vi "SubVI_Camera_Test.vi"(4 "V Width":i32 min=4 max=2048 step=4, 5 "V Offset":i32 min=0 max=0 step=4, 6 "H Width":i32 min=4 max=2048 step=4, 7 "H Offset":i32 min=0 max=0 step=4, 8 "error in":errorcluster, 9 "Exposure Time IN":dbl=0.1 format="%#_13g", 10 "Binning":i32(ring)=1 items=["1x1"=1, "2x2"=2, "4x4"=4], 11 "Menu":T3) -> (0 "error out":errorcluster, 1 "Image":u16[][](graph), 2 "Status":u32, 3 "Temps mesuré ms":u32)   [LabVIEW 2014]
uses:
  Control 1.ctl
  <vilib>/Utility/miscctls.llb/LVMinMaxIncTypeDef.ctl
panel:
  out "Sub Region":T2 {"V Size"."Value" min=0 max=0 step=4; "H Size"."Value" min=0 max=0 step=4; "V Offset"."Value" min=0 max=0 step=4; "H Offset"."Value" min=0 max=0 step=4}
  out "Exposure Time OUT Init S":dbl
  in  "Exposure Time IN Init":dbl=0.1 format="%#_13g"
  out "Exposure Time OUT Init mS":dbl
  out "Exposure Time out":dbl
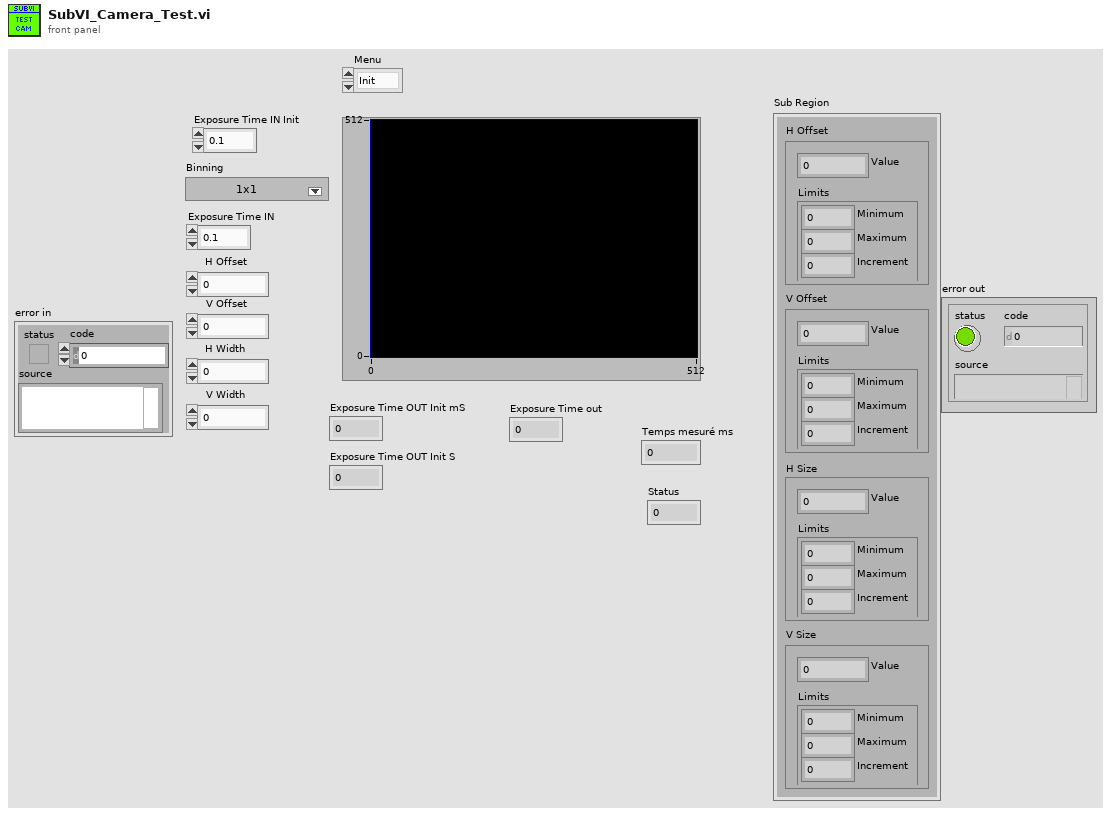
[diagram p1: front panel]
types:
  T1 = typedef "LVMinMaxIncTypeDef.ctl" = cluster{"Minimum":dbl, "Maximum":dbl, "Increment":dbl}
  T2 = cluster{"H Offset":cluster{"Value":i32, "Limits":T1}, "V Offset":cluster{"Value":i32, "Limits":T1}, "H Size":cluster{"Value":i32, "Limits":T1}, "V Size":cluster{"Value":i32, "Limits":T1}}
  T3 = typedef "Control 1.ctl" = enum16{"Init", "Statut", "Binning", "Width", "Exposure Time", "Rep", "Capture", "Stop"}
  T4 = cluster{"H Offset":i32, "V Offset":i32, "H Width":i32, "V Width":i32}
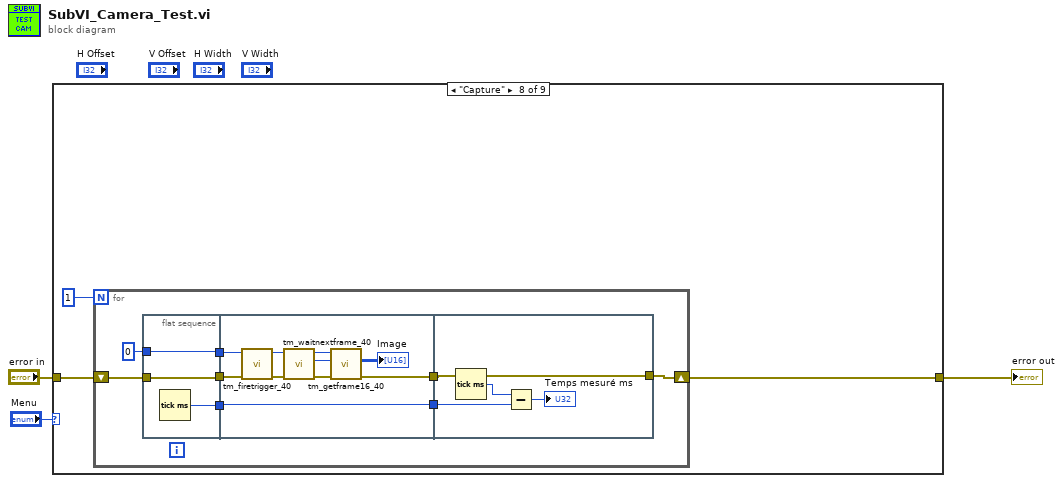
[diagram p0: block diagram]
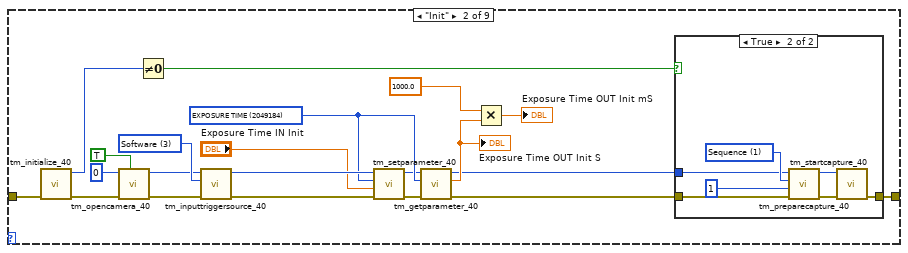
[diagram p3: hidden frame]
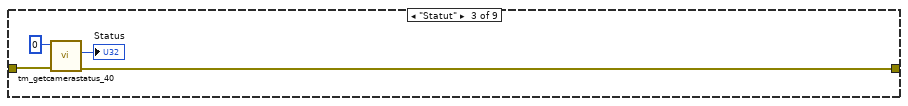
[diagram p5: hidden frame]
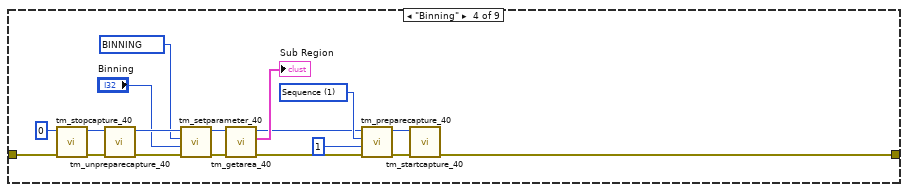
[diagram p6: hidden frame]
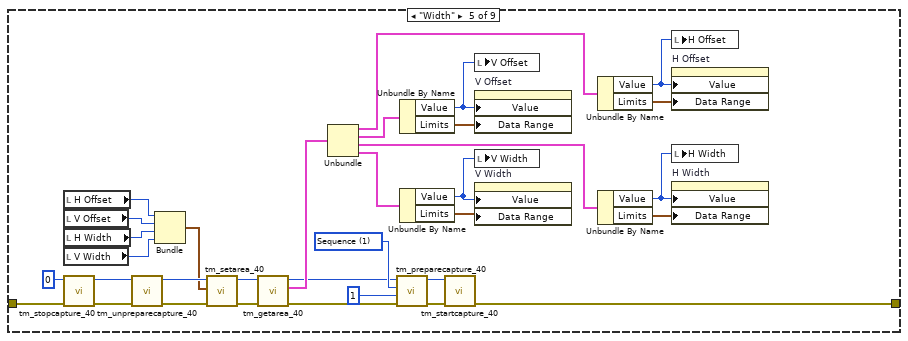
[diagram p7: hidden frame]
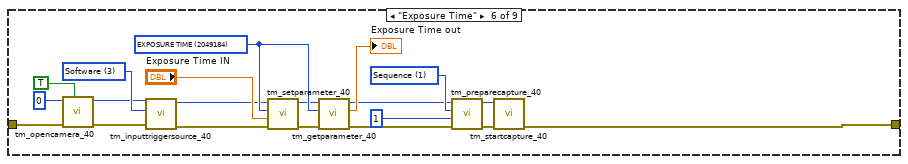
[diagram p8: hidden frame]
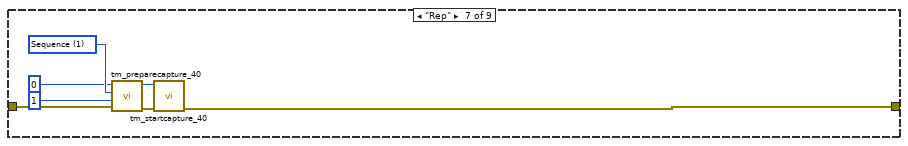
[diagram p9: hidden frame]
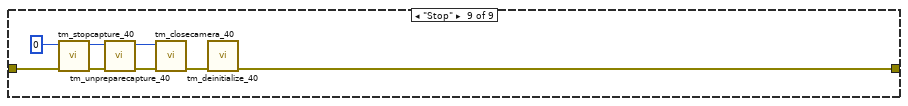
[diagram p10: hidden frame]
diagram:
  n1 = case shown="\"Capture\"" "Menu" {
    tunnel: "error in" -> [w4 w25 w35 w48 w64 w94 w112 w118 w146]
    tunnel: [w4 w5 w37 w38 w57 w98 w111 w117 w144] -> w1
    frame Default {
    }
    frame "Init" {
      w18 = 3 items=["Internal"=1, "External"=2, "Software"=3, "Master Pulse"=4] ("Source")
      w14 = u32 2049184 items=["SENSOR MODE"=4212128, "SENSOR MODE LINE BUNDLE HEIGHT"=4212192, "READOUT DIRECTION"=4211904, "BIT PER CHANNEL"=4342976, "EXPOSURE TIME"=2049184, "CONTRAST GAIN"=3163312, "BINNING"=4215968, "TIMING READOUT TIME"=4223904, "INTERNAL FRAME RATE"=4225952, "INTERNAL FRAME INTERVAL"=4225968, "INTERNAL LINE SPEED"=4226000, "IMAGE WIDTH"=4343200, "IMAGE HEIGHT"=4343216, "IMAGE ROWBYTES"=4343232, "IMAGE FRAMEBYTES"=4343248, "IMAGE PIXEL TYPE"=4343296] ("Parameter")
      n2 = call <userlib>:"tm_initialize_40.vi"("error in (no error)"=w25) -> ("error out"=w22:errorcluster, "Number Of Cameras"=w24:u32)  [unwired: 7 in, 2 out]
      n3 = call <userlib>:"tm_opencamera_40.vi"("Force Open"=TRUE, "error in (no error)"=w22, "Camera Index"=u32 0) -> ("error out"=w10:errorcluster, "Handle out"=w9:u32)  [unwired: 6 in, 1 out]
      n4 = Not Equal To 0?(x=w24) -> (x != 0?=w8:bool)
      n5 = call <userlib>:"tm_inputtriggersource_40.vi"("error in (no error)"=w10, "Source"=w18, "Handle in"=w9) -> ("error out"=w19:errorcluster, "Handle out"=w20:u32)  [unwired: 7 in]
      n6 = call <userlib>:"tm_setparameter_40.vi"("error in (no error)"=w19, "Value in"="Exposure Time IN Init", "Parameter"=w14, "Handle in"=w20) -> ("error out"=w12:errorcluster, "Handle out"=w13:u32)  [unwired: 6 in]
      n7 = call <userlib>:"tm_getparameter_40.vi"("error in (no error)"=w12, "Parameter"=w14, "Handle in"=w13) -> ("error out"=w7:errorcluster, "Value out"=w15:dbl, "Handle out"=w6:u32)  [unwired: 6 in]
      "Exposure Time OUT Init S" <- w15
      n8 = Multiply(x=1000.0, y=w15) -> (x*y=→"Exposure Time OUT Init mS":dbl)
      n9 = case shown="True" w8 {
        tunnel: w7 -> [w26 w28]
        tunnel: w6 -> [_ w29]
        tunnel: [w26 w27] -> w5
        frame False {
        }
        frame True {
          w33 = 1 items=["Snap", "Sequence"] ("Capture mode")
          n10 = call <userlib>:"tm_preparecapture_40.vi"("error in (no error)"=w28, "Frames"=1, "Capture mode"=w33, "Handle in"=w29) -> ("error out"=w31:errorcluster, "Handle out"=w32:u32)  [unwired: 4 in, 2 out]
          n11 = call <userlib>:"tm_startcapture_40.vi"("error in (no error)"=w31, "Handle in"=w32) -> ("error out"=w27:errorcluster)  [unwired: 8 in, 1 out]
        }
      }
    }
    frame "Statut" {
      n12 = call <userlib>:"tm_getcamerastatus_40.vi"("error in (no error)"=w35, "Handle in"=u32 0) -> ("error out"=w37:errorcluster, "Status"=→"Status":i32)  [unwired: 7 in, 1 out]
    }
    frame "Binning" {
      w41 = 1 items=["Snap", "Sequence"] ("Capture mode")
      w52 = u32 4215968 items=["BINNING"=4215968, "BITS PER CHANNEL"=2, "ACTIVE VIEW INDEX"=3, "CCD MODE"=4, "SENSOR MODE"=5, "READOUT MODE"=6, "EXPOSURE TIME"=7, "CONTRAST GAIN"=8, "CONTRAST OFFSET"=9, "LIGHT MODE"=10, "SENSITIVITY"=11, "WHITE BALANCE"=12, "PHOTON IMAGING MODE"=13, "HIGH DYNAMIC RANGE MODE"=14, "TRIGGER SOURCE"=15, "TRIGGER ACTIVE"=16, "TRIGGER MODE"=17, "TRIGGER POLARITY"=18, "TRIGGER GLOBAL EXPOSURE"=19, "FIRST TRIGGER BEHAVIOR"=20, "TRIGGER TIMES"=21, "OUTPUT TRIGGER POLARITY"=22, "OUTPUT TRIGGER DELAY"=23, "OUTPUT TRIGGER PERIOD"=24, "TEMPERATURE"=25, "TEMPERATURE TARGET"=26, "SENSOR COOLER FAN"=27, "MECHANICAL SHUTTER"=28, "BACK FOCUS POSITION"=29, "FRAMEBUNDLE MODE"=30, "FRAMEBUNDLE NUMBER"=31, "LINEBUNDLE HEIGHT"=32, "TRIGGER CONNECTOR"=33, "IMAGE PIXEL TYPE"=34, "OUTPUT TRIGGER KIND"=35, "READOUT DIRECTION"=36, "CHANNEL SYNC"=37] ("Parameter")
      n13 = call <userlib>:"tm_stopcapture_40.vi"("error in (no error)"=w48, "Handle in"=u32 0) -> ("error out"=w50:errorcluster, "Handle out"=w49:u32)  [unwired: 8 in]
      n14 = call <userlib>:"tm_unpreparecapture_40.vi"("error in (no error)"=w50, "Handle in"=w49) -> ("error out"=w51:errorcluster, "Handle out"=w53:u32)  [unwired: 8 in]
      n15 = call <userlib>:"tm_setparameter_40.vi"("error in (no error)"=w51, "Value in"="Binning", "Parameter"=w52, "Handle in"=w53) -> ("error out"=w55:errorcluster, "Handle out"=w54:u32)  [unwired: 6 in]
      n16 = call <userlib>:"tm_getarea_40.vi"("error in (no error)"=w55, "Handle in"=w54) -> ("error out"=w39:errorcluster, "Sub Region"=→"Sub Region":T2, "Handle out"=w40:u32)  [unwired: 7 in]
      n17 = call <userlib>:"tm_preparecapture_40.vi"("error in (no error)"=w39, "Frames"=1, "Capture mode"=w41, "Handle in"=w40) -> ("error out"=w43:errorcluster, "Handle out"=w42:u32)  [unwired: 4 in, 2 out]
      n18 = call <userlib>:"tm_startcapture_40.vi"("error in (no error)"=w43, "Handle in"=w42) -> ("error out"=w38:errorcluster)  [unwired: 8 in, 1 out]
    }
    frame "Width" {
      w62 = 1 items=["Snap", "Sequence"] ("Capture mode")
      n19 = local read "H Offset"() -> (w82:i32)
      n20 = local read "V Offset"() -> (w81:i32)
      n21 = local read "H Width"() -> (w80:i32)
      n22 = local read "V Width"() -> (w79:i32)
      n23 = call <userlib>:"tm_stopcapture_40.vi"("error in (no error)"=w64, "Handle in"=u32 0) -> ("error out"=w84:errorcluster, "Handle out"=w83:u32)  [unwired: 8 in]
      n24 = call <userlib>:"tm_unpreparecapture_40.vi"("error in (no error)"=w84, "Handle in"=w83) -> ("error out"=w86:errorcluster, "Handle out"=w85:u32)  [unwired: 8 in]
      n25 = Bundle("H Offset"=w82, "V Offset"=w81, "H Width"=w80, "V Width"=w79) -> (w78:T4)  [unwired: 1 in]
      n26 = call <userlib>:"tm_setarea_40.vi"("error in (no error)"=w86, "Sub Region"=w78, "Handle in"=w85) -> ("error out"=w88:errorcluster, "Handle out"=w87:u32)  [unwired: 7 in]
      n27 = call <userlib>:"tm_getarea_40.vi"("error in (no error)"=w88, "Handle in"=w87) -> ("error out"=w58:errorcluster, "Sub Region"=w69:T2, "Handle out"=w56:u32)  [unwired: 7 in]
      n28 = Unbundle(w69) -> ("H Offset"=w77:cluster{"Value":i32, "Limits":T1}, "V Offset"=w76:cluster{"Value":i32, "Limits":T1}, "H Size"=w75:cluster{"Value":i32, "Limits":T1}, "V Size"=w74:cluster{"Value":i32, "Limits":T1})
      n29 = call <userlib>:"tm_preparecapture_40.vi"("error in (no error)"=w58, "Frames"=1, "Capture mode"=w62, "Handle in"=w56) -> ("error out"=w60:errorcluster, "Handle out"=w61:u32)  [unwired: 4 in, 2 out]
      n30 = Unbundle By Name(w76) -> ("Value"=w67:i32, "Limits"=w72:T1)
      n31 = Unbundle By Name(w74) -> ("Value"=w65:i32, "Limits"=w70:T1)
      n32 = call <userlib>:"tm_startcapture_40.vi"("error in (no error)"=w60, "Handle in"=w61) -> ("error out"=w57:errorcluster)  [unwired: 8 in, 1 out]
      n33 = local write "V Offset"(w67) -> ()
      n34 = property on="V Offset" class="DigNum (strict)"("Value"=w67, "Data Range"=w72) -> ()  [unwired: 2 in, 2 out]
      n35 = local write "V Width"(w65) -> ()
      n36 = property on="V Width" class="DigNum (strict)"("Value"=w65, "Data Range"=w70) -> ()  [unwired: 2 in, 2 out]
      n37 = Unbundle By Name(w77) -> ("Value"=w68:i32, "Limits"=w73:T1)
      n38 = Unbundle By Name(w75) -> ("Value"=w66:i32, "Limits"=w71:T1)
      n39 = local write "H Offset"(w68) -> ()
      n40 = property on="H Offset" class="DigNum (strict)"("Value"=w68, "Data Range"=w73) -> ()  [unwired: 2 in, 2 out]
      n41 = local write "H Width"(w66) -> ()
      n42 = property on="H Width" class="DigNum (strict)"("Value"=w66, "Data Range"=w71) -> ()  [unwired: 2 in, 2 out]
    }
    frame "Exposure Time" {
      w93 = 3 items=["Internal"=1, "External"=2, "Software"=3, "Master Pulse"=4] ("Source")
      w103 = 1 items=["Snap", "Sequence"] ("Capture mode")
      w108 = u32 2049184 items=["SENSOR MODE"=4212128, "SENSOR MODE LINE BUNDLE HEIGHT"=4212192, "READOUT DIRECTION"=4211904, "BIT PER CHANNEL"=4342976, "EXPOSURE TIME"=2049184, "CONTRAST GAIN"=3163312, "BINNING"=4215968, "TIMING READOUT TIME"=4223904, "INTERNAL FRAME RATE"=4225952, "INTERNAL FRAME INTERVAL"=4225968, "INTERNAL LINE SPEED"=4226000, "IMAGE WIDTH"=4343200, "IMAGE HEIGHT"=4343216, "IMAGE ROWBYTES"=4343232, "IMAGE FRAMEBYTES"=4343248, "IMAGE PIXEL TYPE"=4343296] ("Parameter")
      n43 = call <userlib>:"tm_opencamera_40.vi"("Force Open"=TRUE, "error in (no error)"=w94, "Camera Index"=u32 0) -> ("error out"=w89:errorcluster, "Handle out"=w92:u32)  [unwired: 6 in, 1 out]
      n44 = call <userlib>:"tm_inputtriggersource_40.vi"("error in (no error)"=w89, "Source"=w93, "Handle in"=w92) -> ("error out"=w90:errorcluster, "Handle out"=w91:u32)  [unwired: 7 in]
      n45 = call <userlib>:"tm_setparameter_40.vi"("error in (no error)"=w90, "Value in"="Exposure Time IN", "Parameter"=w108, "Handle in"=w91) -> ("error out"=w106:errorcluster, "Handle out"=w107:u32)  [unwired: 6 in]
      n46 = call <userlib>:"tm_getparameter_40.vi"("error in (no error)"=w106, "Parameter"=w108, "Handle in"=w107) -> ("error out"=w99:errorcluster, "Value out"=→"Exposure Time out":dbl, "Handle out"=w97:u32)  [unwired: 6 in]
      n47 = call <userlib>:"tm_preparecapture_40.vi"("error in (no error)"=w99, "Frames"=1, "Capture mode"=w103, "Handle in"=w97) -> ("error out"=w101:errorcluster, "Handle out"=w100:u32)  [unwired: 4 in, 2 out]
      n48 = call <userlib>:"tm_startcapture_40.vi"("error in (no error)"=w101, "Handle in"=w100) -> ("error out"=w98:errorcluster)  [unwired: 8 in, 1 out]
    }
    frame "Rep" {
      w110 = 1 items=["Snap", "Sequence"] ("Capture mode")
      n49 = call <userlib>:"tm_preparecapture_40.vi"("error in (no error)"=w112, "Frames"=1, "Capture mode"=w110, "Handle in"=u32 0) -> ("error out"=w114:errorcluster, "Handle out"=w115:u32)  [unwired: 4 in, 2 out]
      n50 = call <userlib>:"tm_startcapture_40.vi"("error in (no error)"=w114, "Handle in"=w115) -> ("error out"=w111:errorcluster)  [unwired: 8 in, 1 out]
    }
    frame "Capture" {
      n51 = for {
        N: 1 -> [_]
        shift-right: [w123] -> w117
        shift-left: w118 -> [w119]
        n52 = flat-sequence {
          tunnel: [w129] -> w126
          tunnel: [w128] -> w122
          tunnel: [w127] -> w121
          tunnel: u32 0 ("Handle out") -> [w128]
          tunnel: w119 -> [w127]
          tunnel: [w130] -> w125
          tunnel: [w139] -> w124
          tunnel: w126 -> [w139]
          tunnel: w122 -> [w133]
          tunnel: w121 -> [w132]
          tunnel: [w140] -> w123
          tunnel: w125 -> [w140]
          tunnel: w124 -> [w141]
          frame #0 {
            n53 = Tick Count (ms)() -> (millisecond timer value=w129:u32)
          }
          frame #1 {
            n54 = call <userlib>:"tm_firetrigger_40.vi"("error in (no error)"=w132, "Handle in"=w133) -> ("error out"=w135:errorcluster, "Handle out"=w134:u32)  [unwired: 8 in]
            n55 = call <userlib>:"tm_waitnextframe_40.vi"("error in (no error)"=w135, "Handle in"=w134) -> ("error out"=w138:errorcluster, "Frame Index"=w136:i32, "Handle out"=w137:u32)  [unwired: 6 in, 1 out]
            n56 = call <userlib>:"tm_getframe16_40.vi"("error in (no error)"=w138, "Frame Index"=w136, "Handle in"=w137) -> ("error out"=w130:errorcluster, "Data"=→"Image":u16[][])  [unwired: 5 in, 2 out]
          }
          frame #2 {
            n57 = Tick Count (ms)() -> (millisecond timer value=w142:u32)
            n58 = Subtract(x=w142, y=w141) -> (x-y=→"Temps mesuré ms":u32)
          }
        }
      }
    }
    frame "Stop" {
      n59 = call <userlib>:"tm_stopcapture_40.vi"("error in (no error)"=w146, "Handle in"=u32 0) -> ("error out"=w150:errorcluster, "Handle out"=w149:u32)  [unwired: 8 in]
      n60 = call <userlib>:"tm_unpreparecapture_40.vi"("error in (no error)"=w150, "Handle in"=w149) -> ("error out"=w151:errorcluster, "Handle out"=w148:u32)  [unwired: 8 in]
      n61 = call <userlib>:"tm_closecamera_40.vi"("error in (no error)"=w151, "Handle in"=w148) -> ("error out"=w147:errorcluster)  [unwired: 9 in]
      n62 = call <userlib>:"tm_deinitialize_40.vi"("error in (no error)"=w147) -> ("error out"=w144:errorcluster)  [unwired: 10 in]
    }
  }
  "error out" <- w1
